vi "XYWaveforms.vi"(3 "Microscope Settings":T1={"Mode"=enum."X", "Slit"={"Scanning Mode"=0.0, "Slit Width /%"=0.0}, "Colour"=[], "Exposure/ms"=0.0, "Piezo Position /um"=0.0, "ROI"={"X"={"Start /px"=0.0, "Step /px"=0.0, "Range /px"=0.0}, "Y"={"Start /px"=0.0, "Step /px"=0.0, "Range /px"=0.0}, "Z "={"Start /um"=0.0, "Step/um"=0.0, "Range /um"=0.0}, "T "={"Start /s"=0.0, "Step /s"=1.0, "Range /s"=100.0}}, "Samples per millisecond"=0.0, "Relax/ms"=0.0, "Readout Direction"=0.0, "Trigger Source"=0.0, "Camera Delay /ms"=0.0, "Under Scan /ms"=5.0, "Calibration Coordinates"={"Top Left"=[-4.418670520231216, -0.1592138728323702, 10.0], "Top Right"=[-9.501965317919073, -0.1592138728323702, 10.0], "Bottom Left"=[-4.4508670520231215, 0.0, 0.0], "Bottom Right"=[-9.53757225433526, 0.0, 0.0], "Waveforms"={"Analogue Out"=[], "Digital Out"=[]}}} {"Under Scan /ms" min=0.0 max=10.0 step=0.05; "ROI"."T"."Range /s" min=0.0 max=10.0 step=0.05; "ROI"."T"."Step /s" min=0.0 max=10.0 step=0.05; "ROI"."T"."Start /s" min=0.0 max=10.0 step=0.05; "ROI"."X"."Range /px" min=0.0 max=10.0 step=0.05; "ROI"."X"."Step /px" min=0.0 max=10.0 step=0.05; "ROI"."X"."Start /px" min=0.0 max=10.0 step=0.05; "ROI"."Y"."Range /px" min=0.0 max=10.0 step=0.05; "ROI"."Y"."Step /px" min=0.0 max=10.0 step=0.05; "ROI"."Y"."Start /px" min=0.0 max=10.0 step=0.05; "ROI"."Z"."Range /um" min=0.0 max=10.0 step=0.05; "ROI"."Z"."Step/um" min=0.0 max=10.0 step=0.05; "ROI"."Z"."Start /um" min=0.0 max=10.0 step=0.05; "Colour"."Filter" items=["Empty"=1, ""=2, ""=3, "561"=4, ""=5, "488"=6]; "Camera Delay /ms" min=0.0 max=10.0 step=0.05; "Trigger Source" items=["Internal"=1.0, "External"=2.0]; "Readout Direction" items=["Forward"=1.0, "Backward"=2.0]; "Slit"."Scanning Mode" items=["Full Frame"=1.0, "Slit Scanning"=12.0]; "Piezo Position /um" min=0.0 max=10.0 step=0.05}) -> (0 "Analogue Out":waveform(dbl)[](array[waveform]), 1 "Digital Out":digitalwaveform[](array[waveform]), 2 "dt":dbl)   [LabVIEW 2015]
uses:
  Microscope Settings.ctl
panel:
  out "SignalsGraph":cluster{waveform(dbl)[], digitalwaveform[]}(graph)
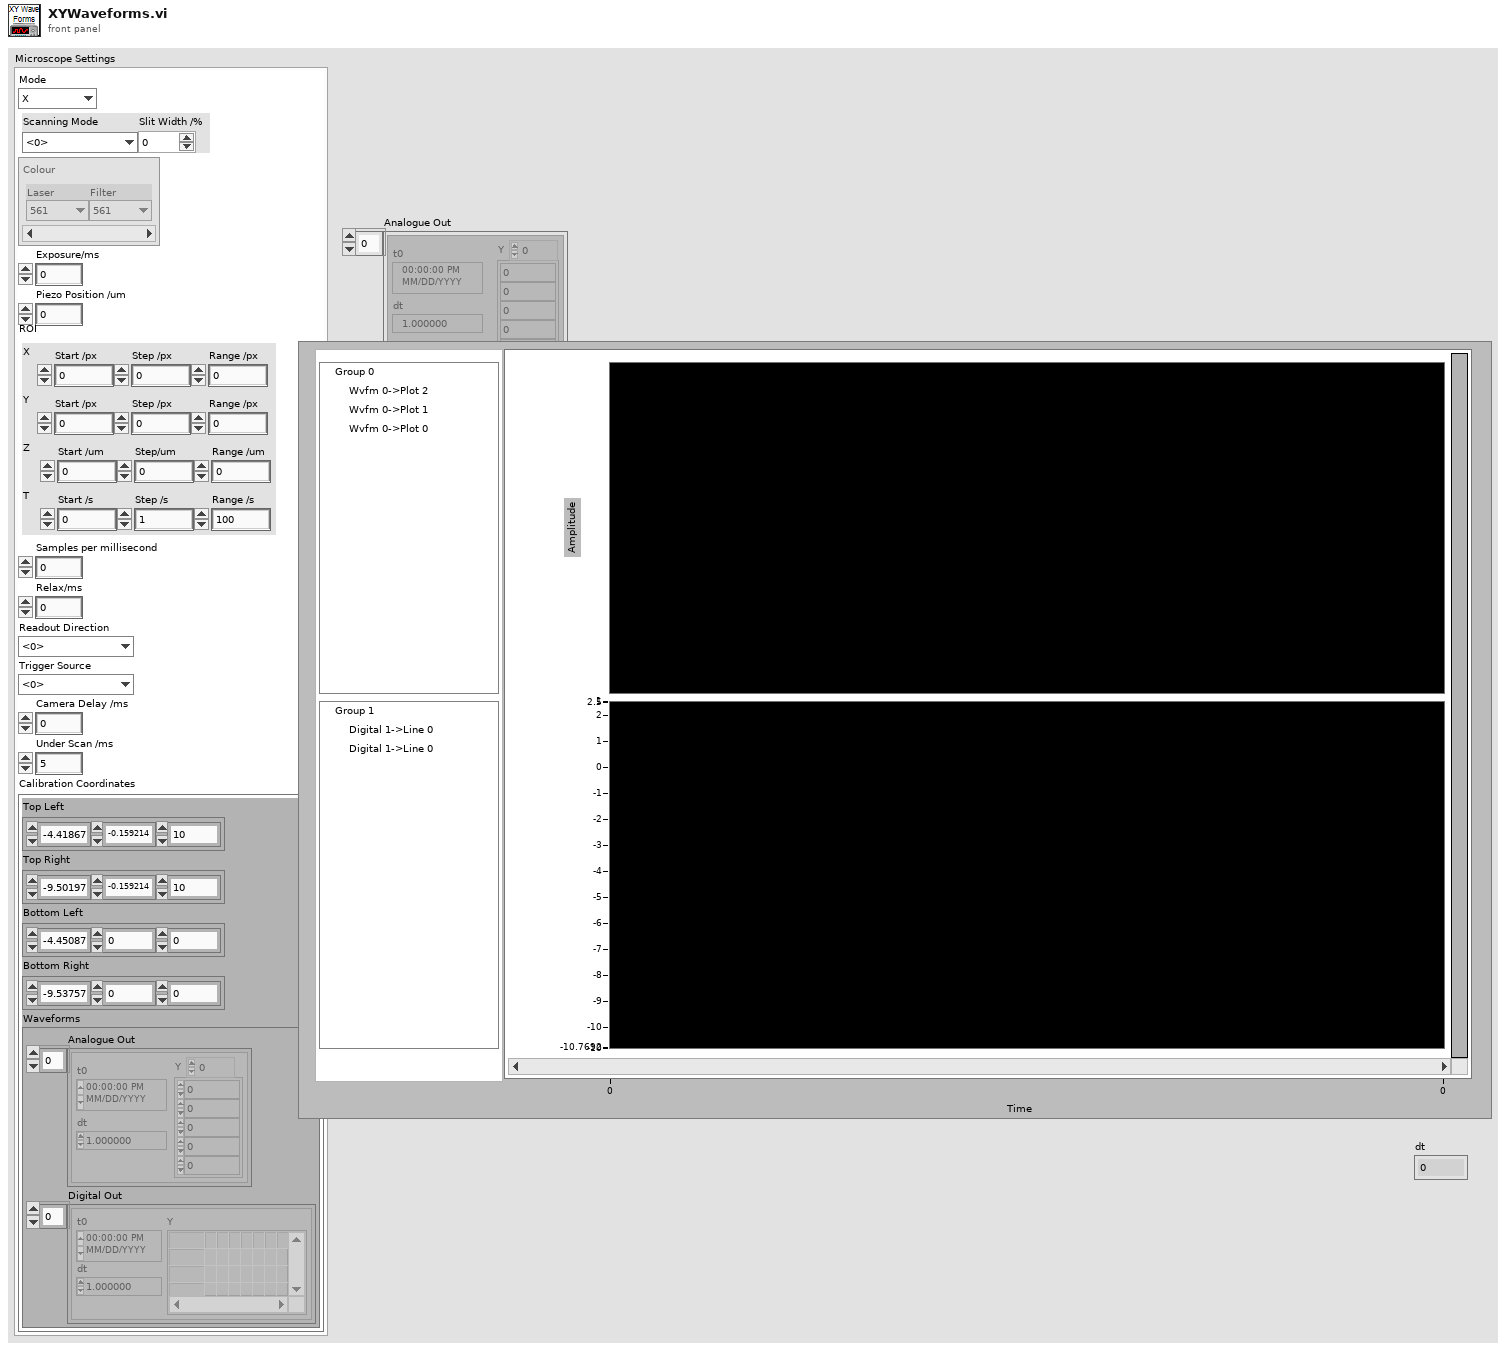
[diagram p1: front panel]
types:
  T1 = typedef "Microscope Settings.ctl" = cluster{"Mode":enum16{"X", "XY", "XYZ", "XYZT", "XYZC", "Tweezers", "Virus"}, "Slit":cluster{"Scanning Mode":dbl, "Slit Width /%":dbl}, "Colour":cluster{"Laser":enum16{"Brightfield", "445", "488", "561", "647"}, "Filter":u16}[], "Exposure/ms":dbl, "Piezo Position /um":dbl, "ROI":cluster{"X":cluster{"Start /px":dbl, "Step /px":dbl, "Range /px":dbl}, "Y":cluster{"Start /px":dbl, "Step /px":dbl, "Range /px":dbl}, "Z ":cluster{"Start /um":dbl, "Step/um":dbl, "Range /um":dbl}, "T ":cluster{"Start /s":dbl, "Step /s":dbl, "Range /s":dbl}}, "Samples per millisecond":dbl, "Relax/ms":dbl, "Readout Direction":dbl, "Trigger Source":dbl, "Camera Delay /ms":dbl, "Under Scan /ms":dbl, "Calibration Coordinates":cluster{"Top Left":dbl[], "Top Right":dbl[], "Bottom Left":dbl[], "Bottom Right":dbl[], "Waveforms":cluster{"Analogue Out":waveform(dbl)[], "Digital Out":digitalwaveform[]}}}
  T2 = cluster{"Laser":enum16{"Brightfield", "445", "488", "561", "647"}, "Filter":u16}[]
  T3 = cluster{"Laser":enum16{"Brightfield", "445", "488", "561", "647"}, "Filter":u16}
  T4 = cluster{"Y Mirror":dbl[], "Z Mirror":dbl[], "Piezo":dbl[], "Camera":dbl[], "Laser":dbl[]}
  T5 = enum16{"Brightfield", "445", "488", "561", "647"}
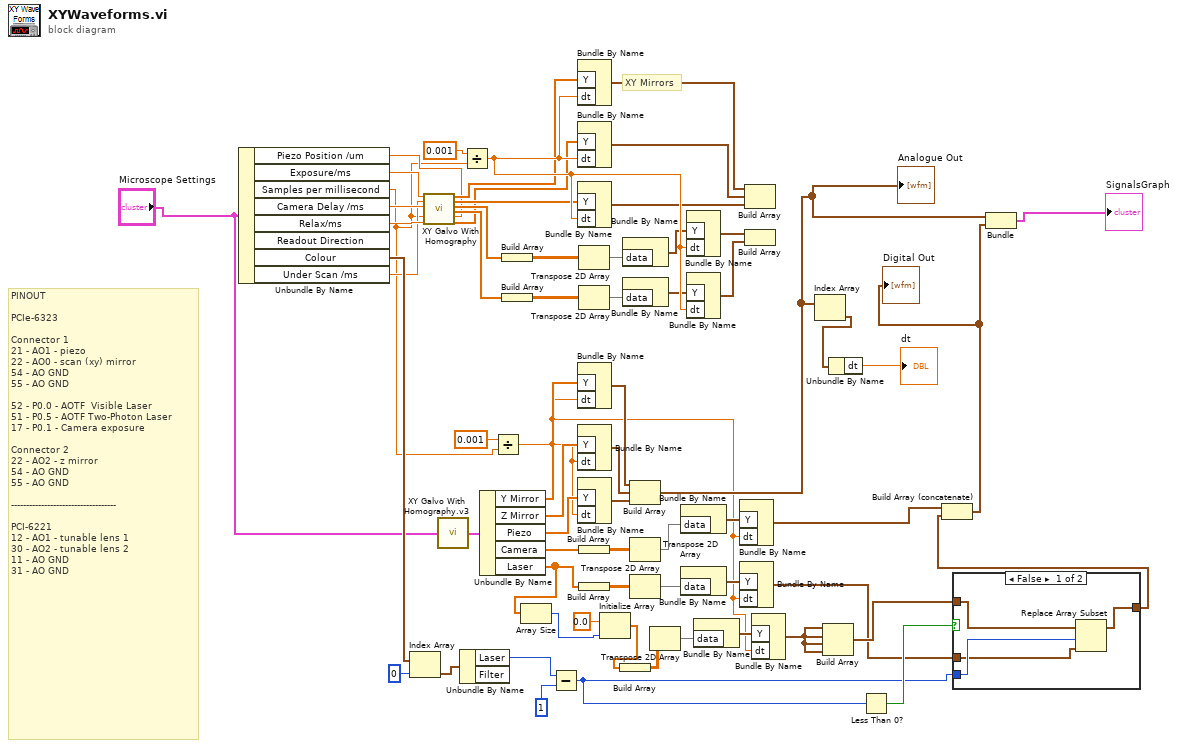
[diagram p0: block diagram]
diagram:
  # "PINOUT\n\nPCIe-6323\n\nConnector 1\n21 - AO1 - piezo\n22 - AO0 - scan (xy) mirror\n54 - AO GND\n55 - AO GND\n\n52 - P0.0 - AOTF  Visible Laser\n51 - P0.5 - AOTF Two-Photon Laser\n17 - P0.1 - Camera exposure\n\nConnector 2\n22 - AO2 - z mirror\n54 - AO GND\n55 - AO GND\n\n-----------------------------------\n\nPCI-6221\n12 - AO1 - tunable lens 1\n30 - AO2 - tunable lens 2\n11 - AO GND\n31 - AO GND"
  # "XY Mirrors"
  n1 = Unbundle By Name("Microscope Settings") -> ("Piezo Position /um"=w41:dbl, "Exposure/ms"=w63:dbl, "Samples per millisecond"=w26:dbl, "Camera Delay /ms"=w62:dbl, "Relax/ms"=w61:dbl, "Colour"=w64:T2, "Under Scan /ms"=w43:dbl)  [unwired: 1 out]
  n2 = Index Array(array=w64, index=0) -> (element=w65:T3)
  n3 = call "XY Galvo With Homography.vi"("Exposure (ms)"=w63, "Underscan /ms"=w43, "Camera Delay /ms"=w62, "Samples /Millisecond"=w26, "Relax (ms)"=w61, "Piezo Position (um)"=w41) -> ("Y Mirror Signal"=w44:dbl[], "Piezo Signal"=w48:dbl[], "Camera Signal"=w58:dbl[], "Laser Signal"=w53:dbl[], "Z Mirror Signal"=w45:dbl[])  [unwired: 9 in]
  n4 = call "XY Galvo With Homography.v3.vi"("Microscope Settings in"="Microscope Settings") -> ("Signals"=w39:T4)
  n5 = Unbundle By Name(w65) -> ("Laser"=w8:T5)  [unwired: 1 out]
  n6 = Divide(x=0.001 ("y"), y=w26) -> (x/y=w59:dbl)
  n7 = Unbundle By Name(w39) -> ("Y Mirror"=w38:dbl[], "Z Mirror"=w37:dbl[], "Piezo"=w35:dbl[], "Camera"=w32:dbl[], "Laser"=w15:dbl[])
  n8 = Divide(x=0.001 ("y"), y=w26) -> (x/y=w1:dbl)
  n9 = Build Array(w58) -> (w57:dbl[][])
  n10 = Build Array(w53) -> (w51:dbl[][])
  n11 = Array Size(array=w15) -> (size(s)=w14:i32)
  n12 = Subtract(x=w8, y=1 ("index")) -> (x-y=w3:i32)
  n13 = Bundle By Name("Y"=w44, "dt"=w59) -> (w47:waveform(dbl))  [unwired: 1 in]
  n14 = Bundle By Name("Y"=w45, "dt"=w59) -> (w46:waveform(dbl))  [unwired: 1 in]
  n15 = Bundle By Name("Y"=w48, "dt"=w59) -> (w49:waveform(dbl))  [unwired: 1 in]
  n16 = Bundle By Name("Y"=w38, "dt"=w1) -> (w21:waveform(dbl))  [unwired: 1 in]
  n17 = Bundle By Name("Y"=w37, "dt"=w1) -> (w36:waveform(dbl))  [unwired: 1 in]
  n18 = Bundle By Name("Y"=w35, "dt"=w1) -> (w34:waveform(dbl))  [unwired: 1 in]
  n19 = Transpose 2D Array(2D array=w57) -> (transposed array=w55:dbl[][])
  n20 = Transpose 2D Array(2D array=w51) -> (transposed array=w54:dbl[][])
  n21 = Build Array(w32) -> (w33:dbl[][])
  n22 = Build Array(w15) -> (w31:dbl[][])
  n23 = Initialize Array(0.0 ("element"), w14) -> (w11:dbl[])
  n24 = Build Array(w11) -> (w10:dbl[][])
  n25 = Bundle By Name("data"=w55) -> (w56:digitaldata)  [unwired: 1 in]
  n26 = Bundle By Name("data"=w54) -> (w52:digitaldata)  [unwired: 1 in]
  n27 = Build Array(w21, w36, w34) -> (w20:waveform(dbl)[])
  "Analogue Out" <- w20
  n28 = Transpose 2D Array(2D array=w33) -> (transposed array=w30:dbl[][])
  n29 = Transpose 2D Array(2D array=w31) -> (transposed array=w29:dbl[][])
  n30 = Transpose 2D Array(2D array=w10) -> (transposed array=w13:dbl[][])
  n31 = Bundle By Name("data"=w30) -> (w28:digitaldata)  [unwired: 1 in]
  n32 = Bundle By Name("data"=w29) -> (w27:digitaldata)  [unwired: 1 in]
  n33 = Bundle By Name("Y"=w56, "dt"=w59) -> (w60:digitalwaveform)  [unwired: 1 in]
  n34 = Bundle By Name("Y"=w52, "dt"=w59) -> (w42:digitalwaveform)  [unwired: 1 in]
  n35 = Bundle By Name("data"=w13) -> (w12:digitaldata)  [unwired: 1 in]
  n36 = Bundle By Name("Y"=w28, "dt"=w1) -> (w24:digitalwaveform)  [unwired: 1 in]
  n37 = Bundle By Name("Y"=w27, "dt"=w1) -> (w4:digitalwaveform)  [unwired: 1 in]
  n38 = Build Array(w47, w46, w49) -> ()  [unwired: 1 out]
  n39 = Build Array(w60, w42) -> ()  [unwired: 1 out]
  n40 = Bundle By Name("Y"=w12, "dt"=w1) -> (w9:digitalwaveform)  [unwired: 1 in]
  n41 = Index Array(array=w20) -> (element=w19:waveform(dbl))  [unwired: 1 in]
  n42 = Build Array(w9, w9, w9, w9) -> (w5:digitalwaveform[])
  n43 = Unbundle By Name(w19) -> ("dt"=→"dt":dbl)
  n44 = Less Than 0?(x=w3) -> (x < 0?=w6:bool)
  n45 = case shown="False" w6 {
    tunnel: w5 -> [w68 w70]
    tunnel: w4 -> [w67 _]
    tunnel: w3 -> [w69 _]
    tunnel: [w66 w70] -> w2
    frame False {
      n46 = Replace Array Subset(array=w68, new element=w67, index=w69) -> (w66:digitalwaveform[])
    }
    frame True {
    }
  }
  n47 = Build Array (concatenate)(w24, w2) -> (w23:digitalwaveform[])
  "Digital Out" <- w23
  n48 = Bundle(w20, w23) -> (→"SignalsGraph":cluster{waveform(dbl)[], digitalwaveform[]})  [unwired: 1 in]
